vi "Yscaling_raw.vi"(6 "Scaling?":u16(ring) items=["Medium", "Large", "Small"], 10 "Y":dbl, 11 "Plane Height (m)":dbl) -> (3 "y scaled (m)":dbl, 4 "Zpos Graph (nm)":T1)   [LabVIEW 2019]
uses:
  GlobalClicksHeight_raw.vi
  <userlib>/HapticSTM/HapticSTM.lvlib
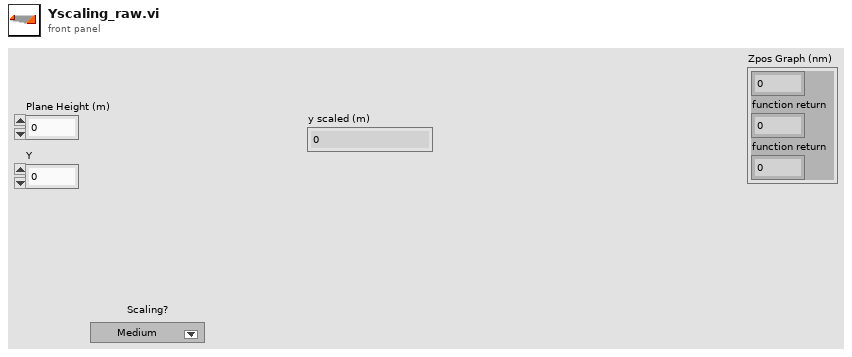
[diagram p1: front panel]
types:
  T1 = cluster{dbl, "function return":dbl, "function return":dbl}
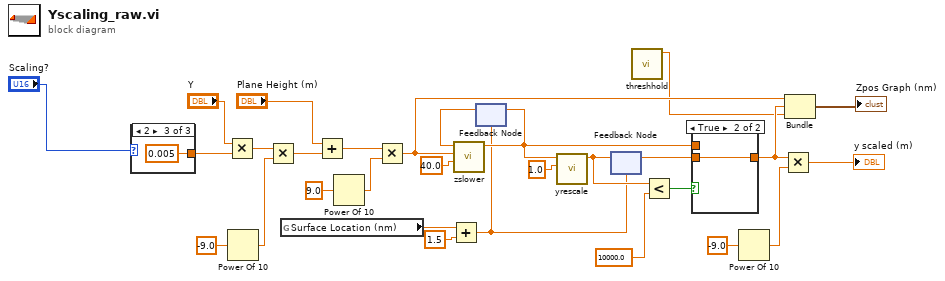
[diagram p0: block diagram]
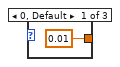
[diagram p2: hidden frame]
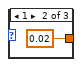
[diagram p3: hidden frame]
diagram:
  n1 = case shown="2" "Scaling?" {
    tunnel: [0.01 ("y") 0.02 ("y") 0.005 ("y")] -> w3
    frame 0, Default {
    }
    frame 1 {
    }
    frame 2 {
    }
  }
  n2 = Multiply(x="Y", y=w3) -> (x*y=w25:dbl)
  n3 = Power Of 10(x=-9.0) -> (10^x=w24:dbl)
  n4 = Multiply(x=w25, y=w24) -> (x*y=w26:dbl)
  n5 = global read "GlobalClicksHeight_raw.vi" "Surface Location (nm)"() -> (w7:dbl)
  n6 = Add(x="Plane Height (m)", y=w26) -> (x+y=w29:dbl)
  n7 = Power Of 10(x=9.0) -> (10^x=w28:dbl)
  n8 = Multiply(x=w29, y=w28) -> (x*y=w10:dbl)
  n9 = Add(x=w7, y=1.5) -> (x+y=w5:dbl)
  n10 = feedback #1(w5) -> (w12:dbl)
  n11 = call <userlib>:"zslower.vi"("maxvel"=40.0, "labview_zpos_write"=w10, "nanonis_zpos_read"=w12) -> ("function return"=w8:dbl)  [unwired: 8 in]
  n12 = feedback-in #1(w8) -> ()
  n13 = call <userlib>:"yrescale.vi"("scalingfactor"=1.0, "ylabview"=w8) -> ("function return"=w9:dbl)  [unwired: 9 in]
  n14 = feedback-in #2(w9) -> ()
  n15 = feedback #2(w5) -> (w14:dbl)
  n16 = call <userlib>:"threshhold.vi"() -> ("function return"=w2:dbl)  [unwired: 11 in]
  n17 = Less?(x=w9, y=10000.0) -> (x < y?=w15:bool)
  n18 = case shown="True" w15 {
    tunnel: [w33 w34] -> w4
    tunnel: w14 -> [_ w34]
    tunnel: w8 -> [w33 _]
    frame False {
    }
    frame True {
    }
  }
  n19 = Power Of 10(x=-9.0) -> (10^x=w19:dbl)
  n20 = Multiply(x=w4, y=w19) -> (x*y=→"y scaled (m)":dbl)
  n21 = Bundle(w10, "function return"=w4, "function return"=w2) -> (→"Zpos Graph (nm)":T1)  [unwired: 1 in]
